vi "Create qeues.vi"(8 "error in (no error)":errorcluster, 9 "name qeue Tx":string, 10 "name qeue Rx":string, 11 "Communication Channel in":refnum<class "Communication Channel.lvclass">) -> (0 "error out":errorcluster, 3 "Communication Channel out":refnum<class "Communication Channel.lvclass">)   [LabVIEW 2018, in "Communication Channel.lvclass"]
uses:
  Communication Channel.lvclass
  RxTx/RxTx.lvclass
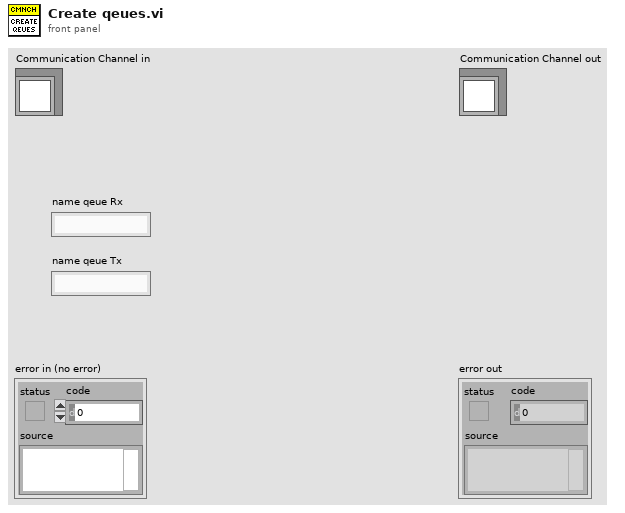
[diagram p1: front panel]
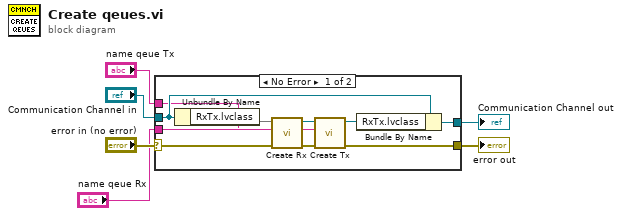
[diagram p0: block diagram]
diagram:
  n1 = case shown="No Error" "error in (no error)" {
    selector: "error in (no error)" -> [w11 w18]
    tunnel: [w9 w18] -> w5
    tunnel: [w15 w17] -> w3
    tunnel: "Communication Channel in" -> [w16 w17]
    tunnel: "name qeue Rx" -> [w8 _]
    tunnel: "name qeue Tx" -> [w7 _]
    frame No Error {
      n2 = Unbundle By Name(w16) -> ("RxTx.lvclass"=w12)
      n3 = call "Create Rx.vi"("error in (no error)"=w11, 10:w8, "RxTx in"=w12) -> ("error out"=w10:errorcluster, "RxTx out"=w13:refnum<class "RxTx.lvclass">)  [unwired: 7 in]
      n4 = call "Create Tx.vi"("error in (no error)"=w10, 10:w7, "RxTx in"=w13) -> ("error out"=w9:errorcluster, "RxTx out"=w14:refnum<class "RxTx.lvclass">)  [unwired: 7 in]
      n5 = Bundle By Name(cluster=w16, "RxTx.lvclass"=w14) -> (w15:refnum<class "Communication Channel.lvclass">)
    }
    frame Error {
    }
  }
  "error out" <- w5
  "Communication Channel out" <- w3
